vi "AutoScan.vi"(8 "error in (no error)":errorcluster, 9 "Autoscan (F: Off)":bool, 10 "Channel (1:1)":u16(ring)=1 items=["1"=1, "2"=2, "3"=3, "4"=4, "5"=5, "6"=6, "7"=7, "8"=8, "9"=9, "10"=10, "11"=11, "12"=12, "13"=13, "14"=14, "15"=15, "16"=16], 11 "VISA resource name":refnum<visa-resource-name>) -> (0 "error out":errorcluster, 3 "VISA resource name out":refnum<visa-resource-name>)   [LabVIEW 2015, in "Lake Shore 372.lvlib"]
doc: "Selects which channel to switch the scanner to and configures the autoscan feature. Functions only when an optional scanner is installed. VI uses <B>SCAN</B> command."
uses:
  Lake Shore 372.lvlib
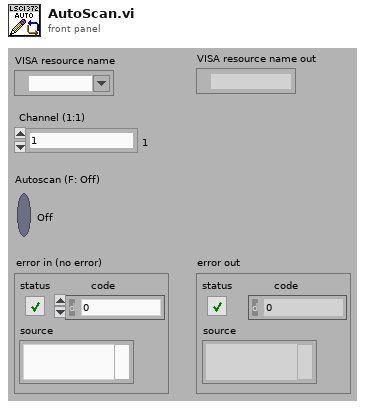
[diagram p1: front panel]
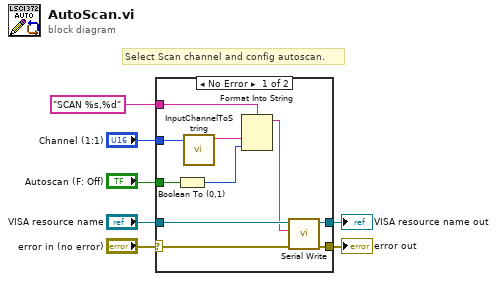
[diagram p0: block diagram]
diagram:
  # "Select Scan channel and config autoscan."
  n1 = case shown="No Error" "error in (no error)" {
    selector: "error in (no error)" -> [w8 w18]
    tunnel: "VISA resource name" -> [w17 w19]
    tunnel: [w16 w18] -> w6
    tunnel: [w15 w19] -> w5
    tunnel: "Autoscan (F: Off)" -> [w14 _]
    tunnel: "SCAN %s,%d" -> [w13 _]
    tunnel: "Channel (1:1)" -> [w10 _]
    frame No Error {
      n2 = Boolean To (0,1)(Boolean=w14) -> (0, 1=w12:i16)
      n3 = call "InputChannelToString.vi"("Channel (1)"=w10) -> ("Channel Str"=w9:string)  [unwired: 10 in]
      n4 = Format Into String(format string=w13, w9, w12) -> (resulting string=w11:string)  [unwired: 2 in, 1 out]
      n5 = call "Serial Write.vi"("error in (no error)"=w8, "Write Buffer (\"\")"=w11, "VISA resource name"=w17) -> ("error out"=w16:errorcluster, "VISA resource name out"=w15:refnum<visa-resource-name>)  [unwired: 6 in, 1 out]
    }
    frame Error {
    }
  }
  "error out" <- w6
  "VISA resource name out" <- w5
